vi "Get area size.vi"(8 "error in (no error)":errorcluster, 10 "Sub Panel":refnum<vi>, 11 "DualScreen in":refnum<class "DualScreen.lvclass">) -> (0 "error out":errorcluster, 2 "Area size (px)":u32, 3 "DualScreen out":refnum<class "DualScreen.lvclass">)   [LabVIEW 2020, in "DualScreen.lvlib" / "DualScreen.lvclass"]
uses:
  DualScreen.lvclass
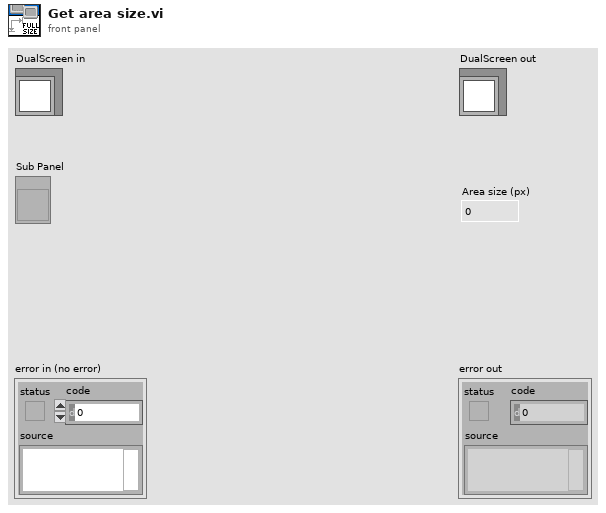
[diagram p1: front panel]
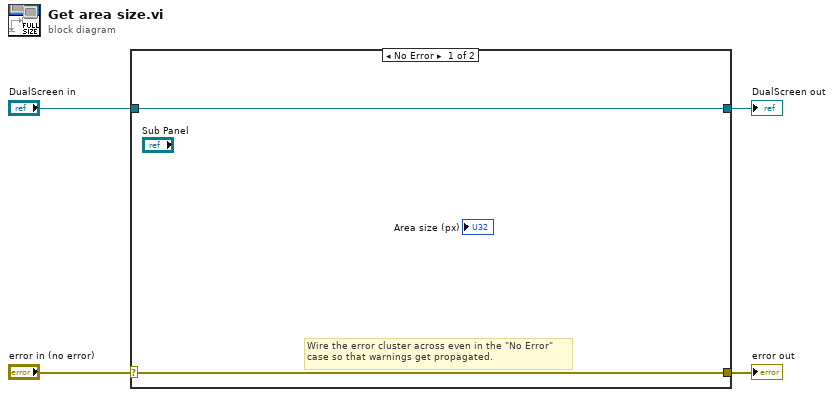
[diagram p0: block diagram]
diagram:
  n1 = case shown="No Error" "error in (no error)" {
    selector: "error in (no error)" -> [w5 w8]
    tunnel: [w5 w8] -> w3
    tunnel: [w6 w7] -> w1
    tunnel: "DualScreen in" -> [w6 w7]
    frame No Error {
      # "Wire the error cluster across even in the \"No Error\"\ncase so that warnings get propagated."
    }
    frame Error {
    }
  }
  "error out" <- w3
  "DualScreen out" <- w1
